vi "ziBW2TC.vi"(1 "Eq BW (F)":bool, 2 "Order (1)":i32=1, 3 "BW (Hz)":dbl) -> (0 "TC (s)":dbl)   [LabVIEW 2018, in "Zurich Instruments LabOne.lvlib"]
doc: "Convert an effective signal bandwidth value and an order value to the required timeconstant per filter order.\n\n<B>Order</B> range: 1 to 8\n<B>Eq BW</B> true: assume BW to be the equivalen-power bandwidht; false: assume BW to be the signal bandwidth"
uses:
  Zurich Instruments LabOne.lvlib
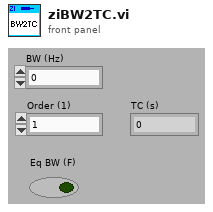
[diagram p1: front panel]
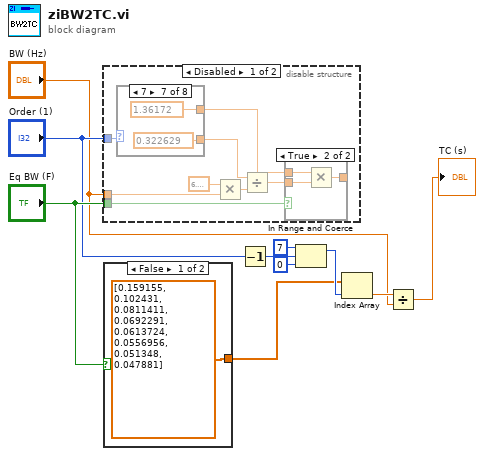
[diagram p0: block diagram]
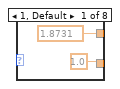
[diagram p3: hidden frame]
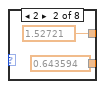
[diagram p4: hidden frame]
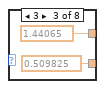
[diagram p5: hidden frame]
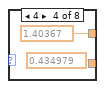
[diagram p6: hidden frame]
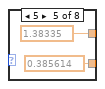
[diagram p7: hidden frame]
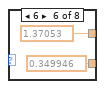
[diagram p8: hidden frame]
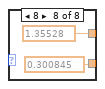
[diagram p9: hidden frame]
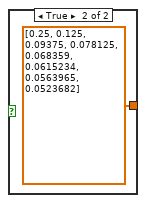
[diagram p11: hidden frame]
diagram:
  n1 = disable-structure shown="Disabled" {
    disable-tunnel: "Eq BW (F)" -> [w13 _]
    disable-tunnel: "Order (1)" -> [w12 _]
    disable-tunnel: "BW (Hz)" -> [w11 _]
    frame Disabled {
      n2 = case shown="7" w12 {
        tunnel: [1.0 ("y") 0.643594 ("y") 0.509825 ("y") 0.434979 ("y") 0.385614 ("y") 0.349946 ("y") 0.322629 ("y") 0.300845 ("y")] -> w16
        tunnel: [1.8731 ("y") 1.52721 ("y") 1.44065 ("y") 1.40367 ("y") 1.38335 ("y") 1.37053 ("y") 1.36172 ("y") 1.35528 ("y")] -> w14
        frame 1, Default {
        }
        frame 2 {
        }
        frame 3 {
        }
        frame 4 {
        }
        frame 5 {
        }
        frame 6 {
        }
        frame 7 {
        }
        frame 8 {
        }
      }
      n3 = Multiply(x=6.283185307179586, y=w11) -> (x*y=w18:dbl)
      n4 = Divide(x=w16, y=w18) -> (x/y=w17:dbl)
      n5 = case shown="True" w13 {
        tunnel: w17 -> [w19 w22]
        tunnel: [w19 w21] -> _
        tunnel: w14 -> [_ w20]
        frame False {
        }
        frame True {
          n6 = Multiply(x=w20, y=w22) -> (x*y=w21:dbl)
        }
      }
    }
    frame Enabled {
    }
  }
  n7 = case shown="False" "Eq BW (F)" {
    tunnel: [dbl[] [0.159155, 0.102431, 0.0811411, 0.0692291, 0.0613724, 0.0556956, 0.051348, 0.047881] dbl[] [0.25, 0.125, 0.09375, 0.078125, 0.068359, 0.0615234, 0.0563965, 0.0523682]] -> w9
    frame False {
    }
    frame True {
    }
  }
  n8 = Decrement(x="Order (1)") -> (x-1=w8:i32)
  n9 = In Range and Coerce(upper limit=7, x=w8, lower limit=0) -> (coerced(x)=w10:i32)  [unwired: 1 out]
  n10 = Index Array(array=w9, index=w10) -> (element=w5:dbl)
  n11 = Divide(x=w5, y="BW (Hz)") -> (x/y=→"TC (s)":dbl)
